vi "Get ProtoParser DLL Directory.vi"() -> (0 "Proto Parser Directory":path)   [LabVIEW 2019, in "gRPC Scripting Tools.lvlib"]
uses:
  gRPC Scripting Tools.lvlib
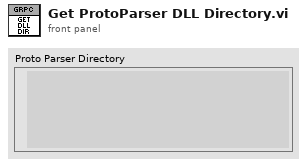
[diagram p1: front panel]
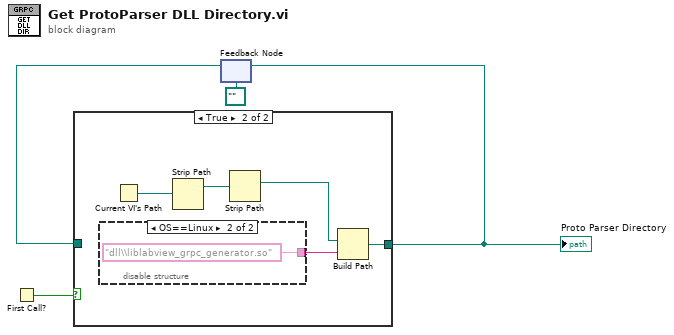
[diagram p0: block diagram]
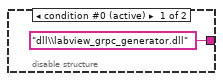
[diagram p3: hidden frame]
diagram:
  n1 = First Call?() -> (First Call?: T/F=w4:bool)
  n2 = feedback #1(path "" ("appended path")) -> (w2:path)
  n3 = case shown="True" w4 {
    tunnel: [w5 w6] -> w3
    tunnel: w2 -> [w5 _]
    frame False {
    }
    frame True {
      n4 = disable-structure shown="OS==Linux" {
        disable-tunnel: ["dll\\labview_grpc_generator.dll" ("name or relative path") "dll\\liblabview_grpc_generator.so" ("name or relative path")] -> w7
        frame condition #0 (active) {
        }
        frame condition #1 {
        }
      }
      n5 = Current VI's Path() -> (path=w8:path)
      n6 = Strip Path(path=w8) -> (stripped path=w9:path)  [unwired: 1 out]
      n7 = Strip Path(path=w9) -> (stripped path=w10:path)  [unwired: 1 out]
      n8 = Build Path(base path=w10, name or relative path=w7) -> (appended path=w6:path)
    }
  }
  "Proto Parser Directory" <- w3
  n9 = feedback-in #1(w3) -> ()
